vi "Read T2114.vi"(8 "error in":errorcluster, 11 "Modbus master in":refnum<class "Modbus Master.lvclass">) -> (0 "error out":errorcluster, 3 "Ambient Pressure, hPa":dbl format="%#_1g")   [LabVIEW 2014, in "T3110 & T2114.lvlib"]
uses:
  T3110 & T2114.lvlib
  <vilib>/NI/Modbus Library/API/Master/Modbus Master.lvclass
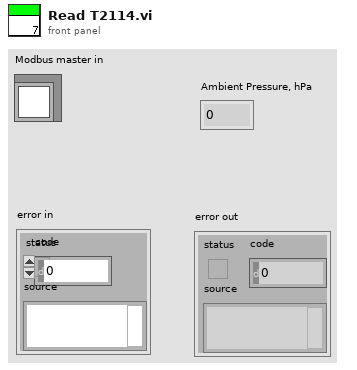
[diagram p1: front panel]
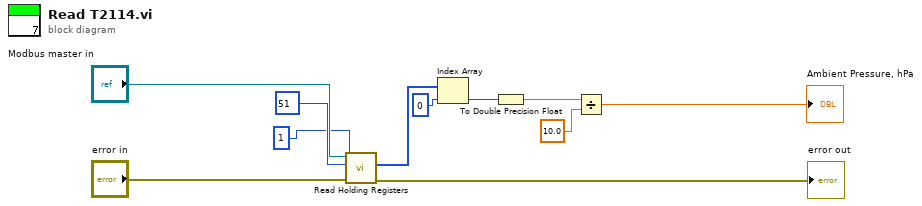
[diagram p0: block diagram]
diagram:
  n1 = call-dynamic "Read Holding Registers.vi"("error in"="error in", "number of inputs"=u16 1, "starting address"=u16 51, "Modbus master in"="Modbus master in") -> ("error out"=→"error out":errorcluster, "register values"=w9:u16[])  [unwired: 5 in, 1 out]
  n2 = Index Array(array=w9, index=0) -> (element=w7:u16)
  n3 = To Double Precision Float(number=w7) -> (double precision float=w6:dbl)
  n4 = Divide(x=w6, y=10.0) -> (x/y=→"Ambient Pressure, hPa":dbl)
